vi "Find_Repeated_measurements.vi"() -> ()   [LabVIEW 2010]
uses:
  Controls/File_Selector_Type.ctl
panel:
  in  "Delete Poor duplicates":bool
  out "Output Log":path=path "/Lacie_20/paulhayden/Documents/Projects/Dapple/Dapple_All_Metadata.tpt"
  in  "Template File":path=path "/Lacie_20/paulhayden/Documents/Projects/Dapple/Dapple_All_Metadata.tpt"
  out "Current file":path=path "/Lacie_20/paulhayden/Desktop/FF_PP/FFID_07_pp.xls"
  in  "Previous Choice":path=path "/Lacie_20/paulhayden/Desktop/FF_PP/FFID_07_pp.xls"
  in  "Search String":string
  in  "At Dialog Prompt Post Process":T1
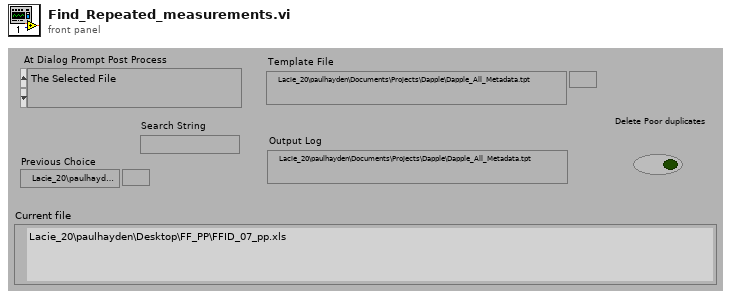
[diagram p1: front panel]
types:
  T1 = typedef "File_Selector_Type.ctl" = enum16{"The Selected File", "The Selected Folder", "Files containing the search string in the selected folder", "All files listed in selected file"}
  T2 = enum32{"existing file", "new file", "new or existing file", "existing dir", "new dir", "new or existing dir", "existing file (use LLBs)", "new file (use LLBs)", "new or existing file (use LLBs)", "new or existing file or directory (use LLBs)"}
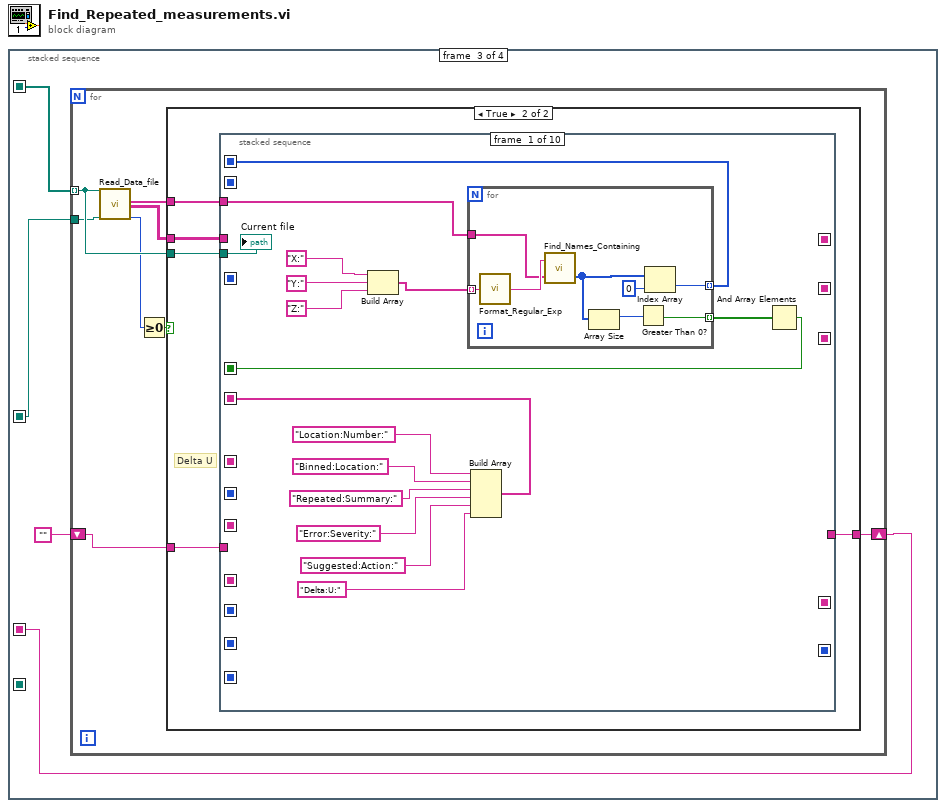
[diagram p0: block diagram]
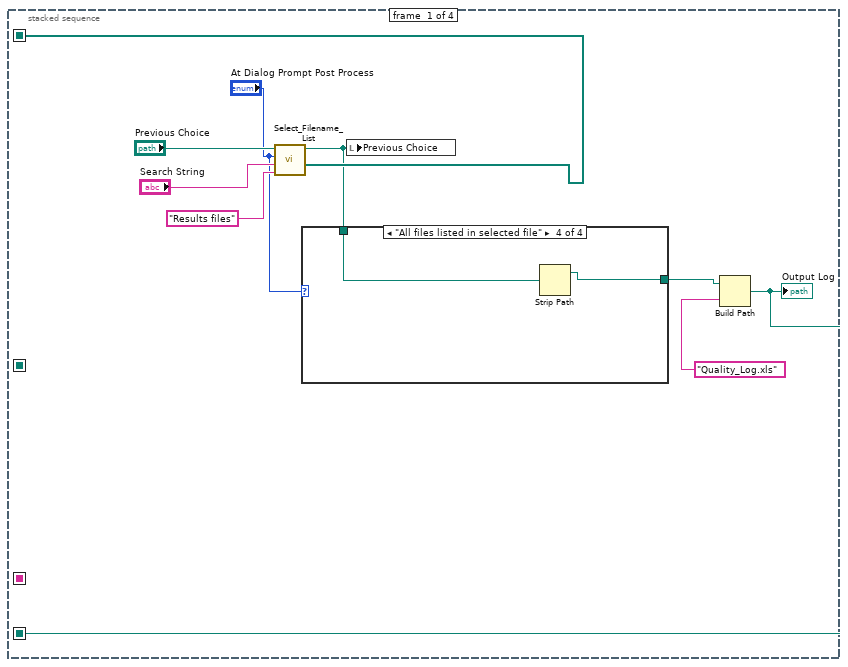
[diagram p2: hidden frame]
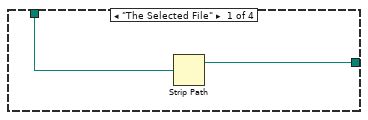
[diagram p3: hidden frame]
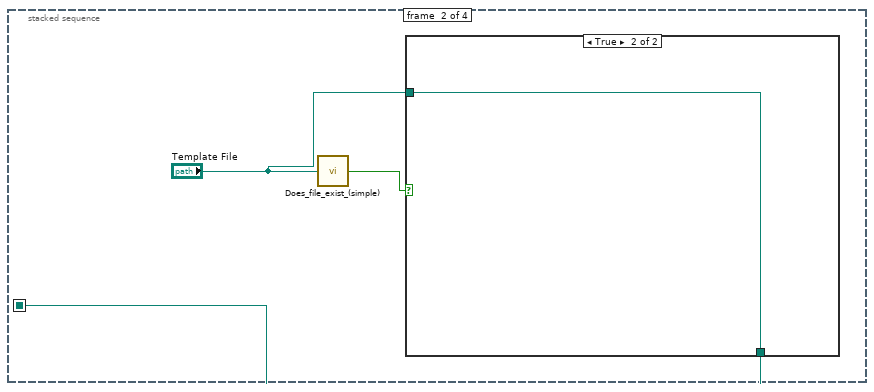
[diagram p6: hidden frame]
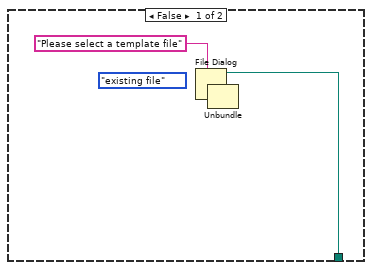
[diagram p7: hidden frame]
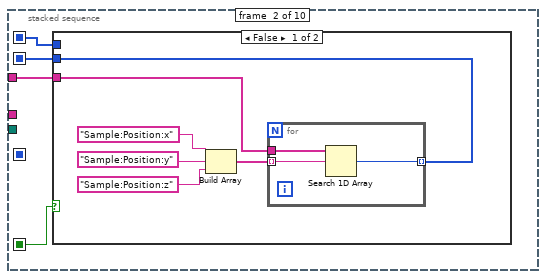
[diagram p9: hidden frame]
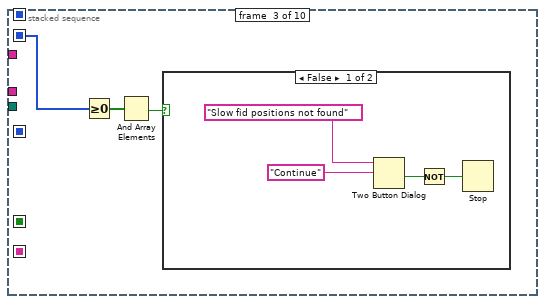
[diagram p11: hidden frame]
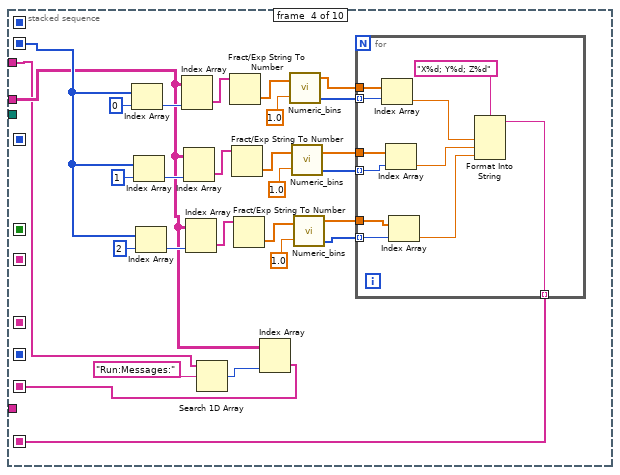
[diagram p13: hidden frame]
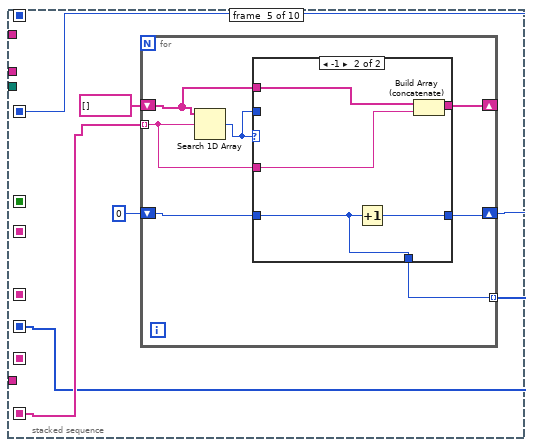
[diagram p14: hidden frame]
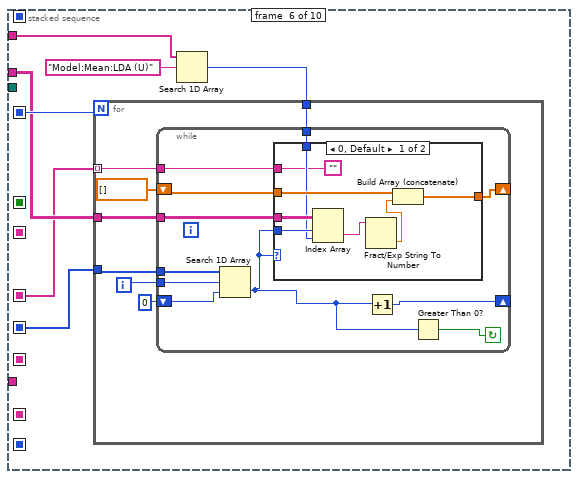
[diagram p16: hidden frame]
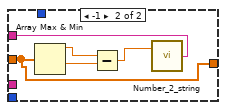
[diagram p17: hidden frame]
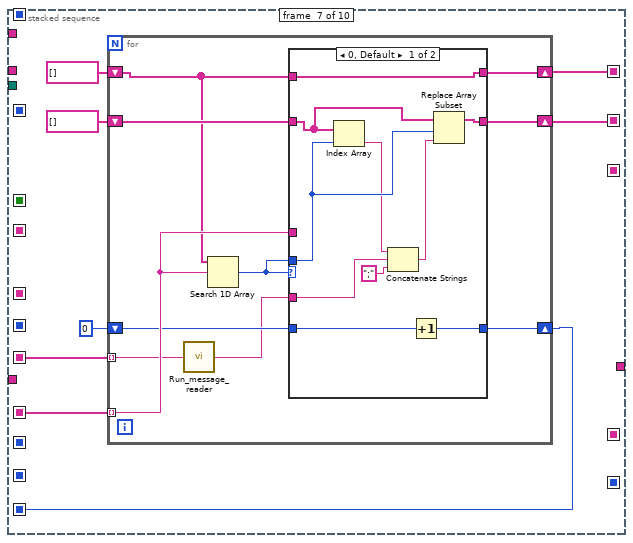
[diagram p18: hidden frame]
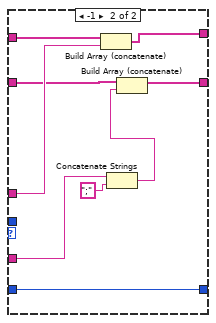
[diagram p19: hidden frame]
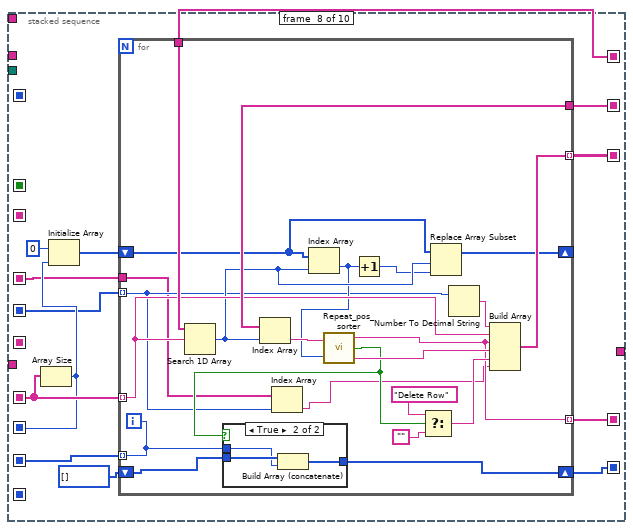
[diagram p20: hidden frame]
diagram:
  n1 = stacked-sequence {
    seq-local: [w6 _ _ _] -> [_ _ w26 _]
    seq-local: [_ _ w24 _] -> [_ _ _ w301]
    seq-local: [w1 _ _ _] -> [_ _ _ w302]
    seq-local: [_ w17 _ _] -> [_ _ w23 _]
    frame #0 {
      n2 = call "Select_Filename_List.vi"("File Type"="Results files", "Search String"="Search String", "At Dialog Prompt Post Process"="At Dialog Prompt Post Process", "Previous Choice"="Previous Choice") -> ("Selected files"=w6:path[], "Choosen path"=w4:path)  [unwired: 2 in, 1 out]
      n3 = case shown="\"All files listed in selected file\"" "At Dialog Prompt Post Process" {
        tunnel: w4 -> [w11 w12 w13 w15]
        tunnel: [w10 w12 w13 w14] -> w3
        frame "The Selected File" {
          n4 = Strip Path(path=w11) -> (stripped path=w10:path)  [unwired: 1 out]
        }
        frame "The Selected Folder" {
        }
        frame "Files containing the search string in the selected folder" {
        }
        frame "All files listed in selected file" {
          n5 = Strip Path(path=w15) -> (stripped path=w14:path)  [unwired: 1 out]
        }
      }
      n6 = local write "Previous Choice"(w4) -> ()
      n7 = Build Path(base path=w3, name or relative path="Quality_Log.xls") -> (appended path=w1:path)
      "Output Log" <- w1
    }
    frame #1 {
      n8 = call "Does_file_exist_(simple).vi"("Pathname"="Template File") -> ("exists?"=w18:bool)
      n9 = case shown="True" w18 {
        tunnel: [w20 w22] -> w17
        tunnel: "Template File" -> [_ w22]
        frame False {
          (unwired) T2."existing file" ("select mode (2)")
          n10 = File Dialog(7:"Please select a template file" ("prompt")) -> (0:w19:errorcluster, 3:w20:path)  [unwired: 6 in, 2 out]
          n11 = Unbundle(w19) -> ()  [unwired: 3 out]
        }
        frame True {
        }
      }
    }
    frame #2 {
      n12 = for {
        tunnel: w26 -> [w32] mode=indexing
        shift-right: [w28] -> w24
        shift-left: "" -> [w29]
        tunnel: w23 -> [w27]
        n13 = call "Read_Data_file.vi"("Results file"=w32, "Template File"=w27) -> ("Ch names Out"=w34:string[], "Channel Values Out"=w33:string[][], "mark after read (chars.)"=w31:i32)  [unwired: 8 in, 7 out]
        n14 = Greater Or Equal To 0?(x=w31) -> (x >= 0?=w30:bool)
        n15 = case shown="True" w30 {
          tunnel: w34 -> [_ w40]
          tunnel: w33 -> [_ w39]
          tunnel: w32 -> [_ w38]
          tunnel: w29 -> [w35 w37]
          tunnel: [w35 w36] -> w28
          frame False {
          }
          frame True {
            # "Delta U"
            n16 = stacked-sequence {
              seq-local: [w50 _ _ _ _ _ _ _ _ _] -> [_ w66 _ _ _ _ _ _ _ _]
              seq-local: [w51 _ _ _ _ _ _ _ _ _] -> [_ _ _ _ _ _ _ _ w268 _]
              seq-local: [_ _ _ _ _ _ _ w230 _ _] -> [_ _ _ _ _ _ _ _ w267 _]
              seq-local: [_ _ _ _ _ _ _ w229 _ _] -> [_ _ _ _ _ _ _ _ w266 _]
              seq-local: [w49 _ _ _ _ _ _ _ _ _] -> [_ w68 _ _ _ _ _ _ _ _]
              seq-local: [_ w67 _ _ _ _ _ _ _ _] -> [_ _ w80 w98 _ _ _ _ _ _]
              seq-local: [_ _ _ w91 _ _ _ _ _ _] -> [_ _ _ _ w129 _ w190 w227 _ _]
              seq-local: [_ _ _ _ _ _ w188 _ _ _] -> [_ _ _ _ _ _ _ w232 _ _]
              seq-local: [_ _ _ _ _ _ w187 _ _ _] -> [_ _ _ _ _ _ _ w231 _ _]
              seq-local: [_ _ _ _ _ _ w185 _ _ _] -> [_ _ _ _ _ _ _ _ w264 _]
              seq-local: [_ _ _ w87 _ _ _ _ _ _] -> [_ _ _ _ _ _ w184 _ _ _]
              seq-local: [_ _ _ _ _ _ _ w225 _ _] -> [_ _ _ _ _ _ _ _ w262 _]
              seq-local: [_ _ _ _ _ _ _ w224 _ _] -> [_ _ _ _ _ _ _ _ w260 _]
              seq-local: [_ _ _ _ _ _ _ w222 _ _] -> [_ _ _ _ _ _ _ _ _ w293]
              seq-local: [_ _ _ _ w126 _ _ _ _ _] -> [_ _ _ _ _ w148 _ w221 _ _]
              seq-local: [_ _ _ _ w125 _ _ _ _ _] -> [_ _ _ _ _ w149 _ _ _ _]
              seq-local: [_ _ _ _ _ w145 _ _ _ _] -> [_ _ _ _ _ _ _ w220 _ _]
              tunnel: w40 -> [w53 w65 _ w86 _ w150 _ _ _ _]
              tunnel: w39 -> [_ _ _ w90 _ w147 _ _ _ _]
              tunnel: w38 -> [w48 _ _ _ _ _ _ _ w269 w292]
              tunnel: w37 -> [_ _ _ _ _ _ _ _ w261 _]
              tunnel: [_ _ _ _ _ _ _ _ w263 _] -> w36
              frame #0 {
                n17 = Build Array("X:", "Y:", "Z:") -> (w41:string[])
                n18 = for {
                  tunnel: w53 -> [w62]
                  tunnel: [w60] -> w50 mode=indexing
                  tunnel: [w57] -> w42 mode=indexing
                  tunnel: w41 -> [w64] mode=indexing
                  n19 = call "Format_Regular_Exp.vi"("Regular expression"=w64) -> ("Case Insensitive for html"=w63:string)
                  n20 = call "Find_Names_Containing.vi"("Ch names"=w62, "String to match"=w63) -> ("Indicies"=w59:i32[])  [unwired: 1 out]
                  n21 = Array Size(array=w59) -> (size(s)=w58:i32)
                  n22 = Greater Than 0?(x=w58) -> (x > 0?=w57:bool)
                  n23 = Index Array(array=w59, index=0) -> (element=w60:i32)
                }
                n24 = Build Array("Location:Number:", "Binned:Location:", "Repeated:Summary:", "Error:Severity:", "Suggested:Action:", "Delta:U:") -> (w51:string[])
                n25 = And Array Elements(Boolean array=w42) -> (logical AND=w49:bool)
                "Current file" <- w48
              }
              frame #1 {
                n26 = case shown="False" w68 {
                  tunnel: w65 -> [w70 _]
                  tunnel: [w69 w78] -> w67
                  tunnel: w66 -> [_ w78]
                  frame False {
                    n27 = Build Array("Sample:Position:x", "Sample:Position:y", "Sample:Position:z") -> (w71:string[])
                    n28 = for {
                      tunnel: w71 -> [w77] mode=indexing
                      tunnel: w70 -> [w76]
                      tunnel: [w75] -> w69 mode=indexing
                      n29 = Search 1D Array(1D array=w76, element=w77) -> (index of element=w75:i32)  [unwired: 1 in]
                    }
                  }
                  frame True {
                  }
                }
              }
              frame #2 {
                n30 = Greater Or Equal To 0?(x=w80) -> (x >= 0?=w81:bool[])
                n31 = And Array Elements(Boolean array=w81) -> (logical AND=w79:bool)
                n32 = case shown="False" w79 {
                  frame False {
                    n33 = Two Button Dialog(message="Slow fid positions not found", 2:"Continue" ("T button name (\"OK\")")) -> (T button?=w83:bool)  [unwired: 1 in]
                    n34 = Not(x=w83) -> (.not. x?=w82:bool)
                    n35 = Stop(stop? (T)=w82) -> ()
                  }
                  frame True {
                  }
                }
              }
              frame #3 {
                n36 = Index Array(array=w98, index=0) -> (element=w112:i32)
                n37 = Index Array(array=w98, index=1) -> (element=w105:i32)
                n38 = Index Array(array=w98, index=2) -> (element=w102:i32)
                n39 = Index Array(array=w90, index (col)=w112) -> (element=w111:string[])  [unwired: 1 in]
                n40 = Index Array(array=w90, index (col)=w105) -> (element=w106:string[])  [unwired: 1 in]
                n41 = Index Array(array=w90, index (col)=w102) -> (element=w101:string[])  [unwired: 1 in]
                n42 = Search 1D Array(1D array=w86, element="Run:Messages:") -> (index of element=w88:i32)  [unwired: 1 in]
                n43 = Fract/Exp String To Number(string=w111) -> (number=w110:dbl[])  [unwired: 3 in, 1 out]
                n44 = Fract/Exp String To Number(string=w106) -> (number=w107:dbl[])  [unwired: 3 in, 1 out]
                n45 = Fract/Exp String To Number(string=w101) -> (number=w100:dbl[])  [unwired: 3 in, 1 out]
                n46 = Index Array(array=w90, index (col)=w88) -> (element=w87:string[])  [unwired: 1 in]
                n47 = call "Numeric_bins.vi"("Values"=w110, "Tolerance"=1.0) -> ("Bin Centres"=w97:dbl[], "Bin Index"=w96:i32[])  [unwired: 1 out]
                n48 = call "Numeric_bins.vi"("Values"=w107, "Tolerance"=1.0) -> ("Bin Centres"=w94:dbl[], "Bin Index"=w92:i32[])  [unwired: 1 out]
                n49 = call "Numeric_bins.vi"("Values"=w100, "Tolerance"=1.0) -> ("Bin Centres"=w95:dbl[], "Bin Index"=w93:i32[])  [unwired: 1 out]
                n50 = for {
                  tunnel: w97 -> [w124]
                  tunnel: w96 -> [w123] mode=indexing
                  tunnel: w95 -> [w122]
                  tunnel: w94 -> [w121]
                  tunnel: w93 -> [w120] mode=indexing
                  tunnel: w92 -> [w119] mode=indexing
                  tunnel: [w114] -> w91 mode=indexing
                  n51 = Index Array(array=w124, index=w123) -> (element=w116:dbl)
                  n52 = Index Array(array=w121, index=w119) -> (element=w117:dbl)
                  n53 = Index Array(array=w122, index=w120) -> (element=w118:dbl)
                  n54 = Format Into String(format string="X%d; Y%d; Z%d", w116, w117, w118) -> (resulting string=w114:string)  [unwired: 2 in, 1 out]
                }
              }
              frame #4 {
                n55 = for {
                  shift-right: [w135] -> _
                  shift-left: string[] [] -> [w136]
                  tunnel: w129 -> [w134] mode=indexing
                  shift-right: [w132] -> w125
                  shift-left: 0 -> [w133]
                  tunnel: [w131] -> w126 mode=indexing
                  n56 = Search 1D Array(1D array=w136, element=w134) -> (index of element=w130:i32)  [unwired: 1 in]
                  n57 = case shown="-1" w130 {
                    tunnel: w136 -> [w137 w144]
                    tunnel: [w137 w143] -> w135
                    tunnel: w134 -> [_ w142]
                    tunnel: w133 -> [w139 w140]
                    tunnel: [w139 w141] -> w132
                    tunnel: [w138 w140] -> w131
                    tunnel: w130 -> [w138 _]
                    frame 0, Default {
                    }
                    frame -1 {
                      n58 = Increment(x=w140) -> (x+1=w141:i32)
                      n59 = Build Array (concatenate)(w144, w142) -> (w143:string[])
                    }
                  }
                }
              }
              frame #5 {
                n60 = Search 1D Array(1D array=w150, element="Model:Mean:LDA (U)") -> (index of element=w146:i32)  [unwired: 1 in]
                n61 = for {
                  N: w149 -> [_]
                  tunnel: w148 -> [w158]
                  tunnel: w147 -> [w155]
                  tunnel: w146 -> [w154]
                  tunnel: [w152] -> w145 mode=indexing
                  i -> [w157]
                  n62 = while {
                    tunnel: w158 -> [w169]
                    tunnel: w157 -> [w168]
                    shift-right: [w160] -> _
                    shift-left: 0 -> [w167]
                    shift-right: [w162] -> _
                    shift-left: dbl[] [] -> [w165]
                    tunnel: w155 -> [w164]
                    tunnel: w154 -> [w163]
                    tunnel: [w161] -> w152
                    stop <- w166 continue-if-true
                    n63 = Search 1D Array(1D array=w169, element=w168, start index (0)=w167) -> (index of element=w159:i32)
                    n64 = case shown="0, Default" w159 {
                      tunnel: w165 -> [w177 w180]
                      tunnel: w164 -> [w176 _]
                      tunnel: w159 -> [w175 _]
                      tunnel: w163 -> [w174 _]
                      tunnel: [w173 w180] -> w162
                      tunnel: ["" w178] -> w161
                      frame 0, Default {
                        n65 = Index Array(array=w176, index (row)=w175, index (col)=w174) -> (element=w172:string)
                        n66 = Fract/Exp String To Number(string=w172) -> (number=w171:dbl)  [unwired: 3 in, 1 out]
                        n67 = Build Array (concatenate)(w177, w171) -> (w173:dbl[])
                      }
                      frame -1 {
                        n68 = Array Max & Min(array=w180) -> (max value=w182:dbl, min value=w181:dbl)  [unwired: 2 out]
                        n69 = Subtract(x=w182, y=w181) -> (x-y=w179:dbl)
                        n70 = call "Number_2_string.vi"("number"=w179) -> ("String"=w178:string)  [unwired: 1 in]
                      }
                    }
                    n71 = Increment(x=w159) -> (x+1=w160:i32)
                    n72 = Greater Than 0?(x=w159) -> (x > 0?=w166:bool)
                  }
                }
              }
              frame #6 {
                n73 = for {
                  shift-right: [w200] -> w188
                  shift-left: string[] [] -> [w196]
                  shift-right: [w197] -> w187
                  shift-left: string[] [] -> [w198]
                  tunnel: w190 -> [w199] mode=indexing
                  shift-right: [w193] -> w185
                  shift-left: 0 -> [w194]
                  tunnel: w184 -> [w192] mode=indexing
                  n74 = call "Run_message_reader.vi"("Run Message"=w192) -> ("Error Severity"=w191:string)
                  n75 = Search 1D Array(1D array=w196, element=w199) -> (index of element=w195:i32)  [unwired: 1 in]
                  n76 = case shown="0, Default" w195 {
                    tunnel: w196 -> [w207 w219]
                    tunnel: [w207 w218] -> w200
                    tunnel: w199 -> [_ w217]
                    tunnel: w198 -> [w210 w216]
                    tunnel: [w208 w215] -> w197
                    tunnel: w195 -> [w209 _]
                    tunnel: w194 -> [w206 w214]
                    tunnel: [w205 w214] -> w193
                    tunnel: w191 -> [w203 w213]
                    frame 0, Default {
                      n77 = Index Array(array=w210, index=w209) -> (element=w201:string)
                      n78 = Concatenate Strings(w201, w203, ";" ("string")) -> (w202:string)
                      n79 = Increment(x=w206) -> (x+1=w205:i32)
                      n80 = Replace Array Subset(array=w210, new element=w202, index=w209) -> (w208:string[])
                    }
                    frame -1 {
                      n81 = Build Array (concatenate)(w219, w217) -> (w218:string[])
                      n82 = Concatenate Strings(w213, ";" ("string")) -> (w211:string)
                      n83 = Build Array (concatenate)(w216, w211) -> (w215:string[])
                    }
                  }
                }
              }
              frame #7 {
                n84 = Array Size(array=w227) -> (size(s)=w224:i32)
                n85 = Initialize Array(0 ("element"), w224) -> (w226:i32[])
                n86 = for {
                  tunnel: w232 -> [w255]
                  tunnel: w227 -> [w252] mode=indexing
                  tunnel: w231 -> [w254]
                  tunnel: [w253] -> w230 mode=indexing
                  tunnel: [w236] -> w229 mode=indexing
                  shift-right: [w249] -> _
                  shift-left: w226 -> [w250]
                  tunnel: [w241] -> w225 mode=indexing
                  shift-right: [w238] -> w222
                  shift-left: i32[] [] -> [w239]
                  tunnel: w221 -> [w235] mode=indexing
                  tunnel: w220 -> [w234]
                  i -> [w236]
                  n87 = Search 1D Array(1D array=w255, element=w252) -> (index of element=w251:i32)  [unwired: 1 in]
                  n88 = Index Array(array=w254, index=w251) -> (element=w247:string)
                  n89 = Index Array(array=w234, index=w235) -> (element=w233:string)
                  n90 = Index Array(array=w250, index=w251) -> (element=w246:i32)
                  n91 = call "Repeat_pos_sorter.vi"("Concatenated Run Messages"=w247, "Index"=w246) -> ("Decision"=w241:string, "Delete Row"=w240:bool, "Error Severity"=w242:string)
                  n92 = case shown="True" w240 {
                    tunnel: w239 -> [w256 w259]
                    tunnel: w236 -> [_ w258]
                    tunnel: [w256 w257] -> w238
                    frame False {
                    }
                    frame True {
                      n93 = Build Array (concatenate)(w259, w258) -> (w257:i32[])
                    }
                  }
                  n94 = Increment(x=w246) -> (x+1=w248:i32)
                  n95 = Select(t="Delete Row", s=w240, f="") -> (s? t:f=w243:string)
                  n96 = Replace Array Subset(array=w250, new element=w248, index=w251) -> (w249:i32[])
                  n97 = Number To Decimal String(number=w235) -> (decimal integer string=w237:string)  [unwired: 1 in]
                  n98 = Build Array(w237, w252, w241, w242, w243, w233) -> (w253:string[])
                }
              }
              frame #8 {
                n99 = Greater Than 0?(x=w264) -> (x > 0?=w265:bool)
                n100 = case shown="True" w265 {
                  tunnel: w269 -> [_ w281]
                  tunnel: w268 -> [_ w285]
                  tunnel: w267 -> [_ w284]
                  tunnel: w266 -> [_ w283]
                  tunnel: w264 -> [_ w272]
                  tunnel: [w270 w279] -> w263
                  tunnel: w262 -> [_ w276]
                  tunnel: w261 -> [w270 w275]
                  tunnel: w260 -> [_ w271]
                  frame False {
                  }
                  frame True {
                    w282 = FALSE  # Value  Constant?
                    n101 = call "Analyse_string_array.vi"("String array"=w276) -> ("Unique strings"=w277:string[], "Frequency"=w278:i32[])  [unwired: 1 in]
                    n102 = for {
                      tunnel: w278 -> [w290] mode=indexing
                      shift-right: [w286] -> w273
                      shift-left: "" -> [w287]
                      tunnel: w277 -> [w288] mode=indexing
                      n103 = Format Into String(format string="%s (%d)\t", initial string=w287, w288, w290) -> (resulting string=w286:string)  [unwired: 1 in, 1 out]
                    }
                    n104 = call "Add_Update_Values_sub.vi"("Value  Constant?"=w282, "Selected Rows"=w283, "New Values In"=w284, "New Chs In"=w285, "Filename"=w281) -> ()  [unwired: 6 in, 1 out]
                    n105 = Format Into String(format string="%s\t%d\t%d\t%s\r", initial string=w275, w281, w271, w272, w273) -> (resulting string=w279:string)  [unwired: 1 in, 1 out]
                  }
                }
              }
              frame #9 {
                n106 = case shown="False" "Delete Poor duplicates" {
                  tunnel: w293 -> [_ w296]
                  tunnel: w292 -> [_ w297]
                  frame False {
                  }
                  frame True {
                    n107 = Array Size(array=w296) -> (size(s)=w295:i32)
                    n108 = Greater Than 0?(x=w295) -> (x > 0?=w294:bool)
                    n109 = case shown="True" w294 {
                      tunnel: w297 -> [_ w299]
                      tunnel: w296 -> [_ w298]
                      frame False {
                      }
                      frame True {
                        n110 = call "Delete_unwanted_rows.vi"("Selected Rows"=w298, "Filename"=w299) -> ()  [unwired: 1 in]
                      }
                    }
                  }
                }
              }
            }
          }
        }
      }
    }
    frame #3 {
      n111 = Empty String/Path?(string/path=w301) -> (empty?=w300:bool)
      n112 = case shown="False" w300 {
        tunnel: w302 -> [w306 _]
        tunnel: w301 -> [w304 _]
        frame False {
          n113 = call "Does_file_exist_(simple).vi"("Pathname"=w306) -> ("exists?"=w305:bool)
          n114 = case shown="True" w305 {
            tunnel: w304 -> [w310 w319]
            tunnel: [w308 w319] -> w303
            frame False {
              n115 = Build Array("Results:Filename:", "Number of:Row in File:", "Number of:Dulicated Rows:", "Duplication:Information") -> (w314:string[])
              n116 = call "Ch_names_to_rows.vi"("Channel Names"=w314) -> ("3 Row names"=w312:string[][])
              n117 = Array To Spreadsheet String(array=w312, 3:"%s" ("format string")) -> (spreadsheet string=w311:string)  [unwired: 1 in]
              n118 = Concatenate Strings(w311, "\r", w310) -> (w308:string)
            }
            frame True {
            }
          }
          n119 = call "Write_Characters_To_File.vi"("file path (dialog if empty)"=w306, "character string"=w303, "append to file? (new file:F)"=TRUE) -> ()  [unwired: 5 in, 1 out]
        }
        frame True {
        }
      }
    }
  }
